vi "terminate.vi"(8 "error in (no error)":errorcluster) -> (0 "error out":errorcluster)   [LabVIEW 2010, in "CPUmonitor.lvclass"]
uses:
  CPUmonitor.lvclass
  class_data.vi
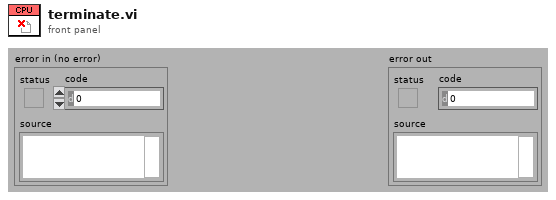
[diagram p1: front panel]
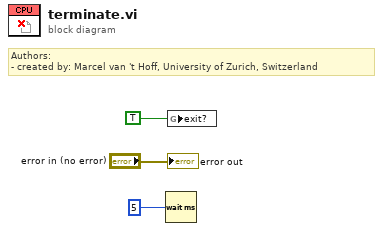
[diagram p0: block diagram]
diagram:
  # "Authors: \n- created by: Marcel van 't Hoff, University of Zurich, Switzerland"
  n1 = Wait (ms)(milliseconds to wait=u32 5) -> ()  [unwired: 1 out]
  n2 = global write "class_data.vi" "exit?"(TRUE ("exit?")) -> ()
  "error out" <- "error in (no error)"
